vi "SetValueByArrayIndex.vi"(0 "VI Reference In":refnum<vi>, 2 "delimiter (>>)":string=">>", 5 "Control Path":string, 7 "Index Array":i32[](array[numeric]), 11 "Error In":errorcluster) -> (4 "VI Reference Out":refnum<vi>, 15 "Error Out":errorcluster)   [LabVIEW 2016, in "Drona.lvlib" / "ControlValue.lvlib" / "StimulusMCListbox.lvlib"]
doc: "Sets value(signaling) for the multi select multi column listbox control whose index values are specified. \n\nThe input control name is given as a string , incase of path, use delimiters inbetween the path."
uses:
  StimulusMCListbox.lvlib
  <vilib>/Utility/error.llb/Error Cluster From Error Code.vi
  <vilib>/ErrorRing/Error Ring.xnode
  Drona.lvlib
  Get/GetControlRef/GetControlRef.lvlib
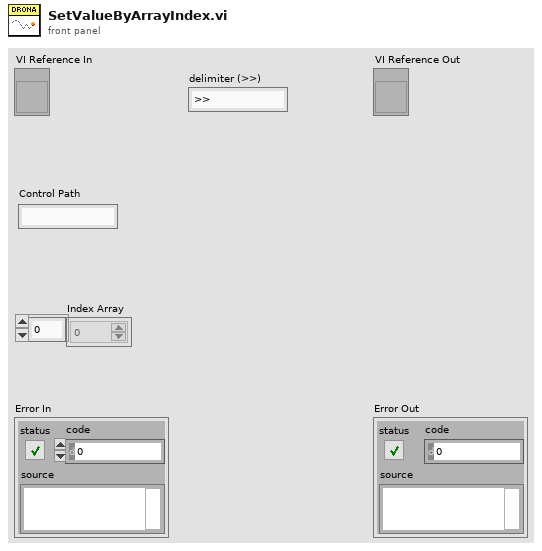
[diagram p1: front panel]
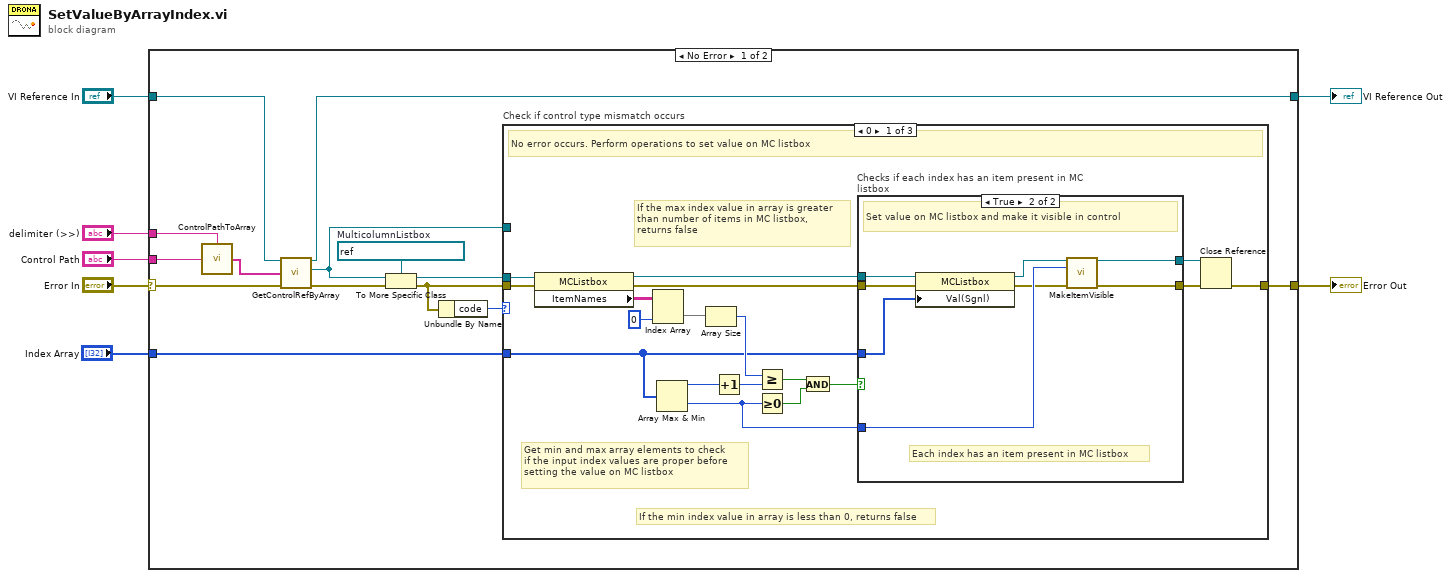
[diagram p0: block diagram]
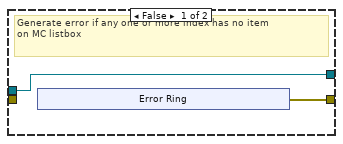
[diagram p2: hidden frame]
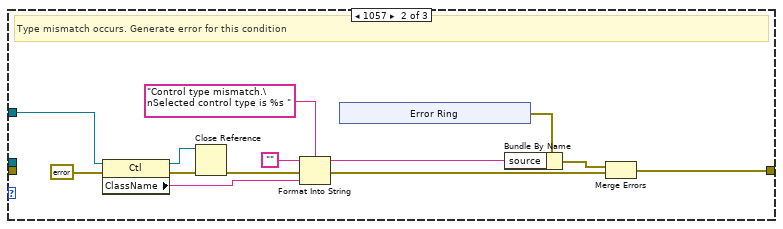
[diagram p3: hidden frame]
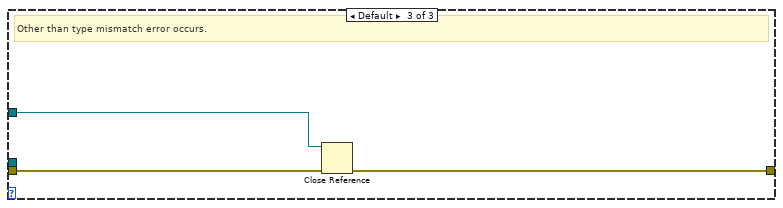
[diagram p4: hidden frame]
diagram:
  n1 = case shown="No Error" "Error In" {
    selector: "Error In" -> [w16 w77]
    tunnel: [w17 w77] -> w6
    tunnel: "VI Reference In" -> [w14 w76]
    tunnel: "Control Path" -> [w20 _]
    tunnel: "Index Array" -> [w11 _]
    tunnel: [w13 w76] -> w2
    tunnel: "delimiter (>>)" -> [w19 _]
    frame No Error {
      w21 = refnum<vi> refnum  # MulticolumnListbox
      n2 = call "ControlPathToArray.vi"("Control Name"=w20, "delimiter (>>)"=w19) -> ("Control Path"=w15:string[])
      n3 = call "GetControlRefByArray.vi"("VI Reference In"=w14, "Control Path"=w15, "error In"=w16) -> ("VI Reference Out"=w13:refnum<vi>, "Ctl Refnum"=w8:refnum<vi>, "error out"=w12:errorcluster)  [unwired: 10 in]
      n4 = To More Specific Class(target class=w21, reference=w8, error in=w12) -> (specific class reference=w18:refnum<vi>, error out=w10:errorcluster)
      n5 = Unbundle By Name(w10) -> ("code"=w9:i32)
      n6 = case "Check if control type mismatch occurs" shown="0" w9 {
        tunnel: w10 -> [w39 _ w75]
        tunnel: w18 -> [w35 _ _]
        tunnel: [w31 w55 w74] -> w17
        tunnel: w11 -> [w26 _ _]
        tunnel: w8 -> [_ w56 w73]
        frame 0 {
          # "If the min index value in array is less than 0, returns false"
          # "If the max index value in array is greater \nthan number of items in MC listbox, \nreturns false"
          # "Get min and max array elements to check \nif the input index values are proper before \nsetting the value on MC listbox"
          # "No error occurs. Perform operations to set value on MC listbox"
          n7 = property class="MCListbox"(reference=w35, error in=w39) -> (reference out=w34:refnum<vi>, error out=w36:errorcluster, "ItemNames"=w24:string[][])
          n8 = Index Array(array=w24, index (col)=0 ("disabled index (col)")) -> (element=w22:string[])  [unwired: 1 in]
          n9 = Array Max & Min(array=w26) -> (max value=w30:i32, min value=w28:i32)  [unwired: 2 out]
          n10 = Array Size(array=w22) -> (size(s)=w33:i32)
          n11 = Increment(x=w30) -> (x+1=w29:i32)
          n12 = Greater Or Equal?(x=w33, y=w29) -> (x >= y?=w27:bool)
          n13 = Greater Or Equal To 0?(x=w28) -> (x >= 0?=w25:bool)
          n14 = And(x=w27, y=w25) -> (x .and. y?=w32:bool)
          n15 = case "Checks if each index has an item present in MC listbox" shown="True" w32 {
            tunnel: [w40 w54] -> w38
            tunnel: [w41 w53] -> w37
            tunnel: w28 -> [_ w52]
            tunnel: w36 -> [_ w51]
            tunnel: w34 -> [w41 w49]
            tunnel: w26 -> [_ w48]
            frame False {
              # "Generate error if any one or more index has no item \non MC listbox"
              n16 = xnode "Error Ring"() -> ("error out"=w40:errorcluster)
            }
            frame True {
              # "Each index has an item present in MC listbox"
              # "Set value on MC listbox and make it visible in control"
              n17 = property class="MCListbox"(reference=w49, error in=w51, "Val(Sgnl)"=w48) -> (reference out=w47:refnum<vi>, error out=w50:errorcluster)
              n18 = call "MakeItemVisible.vi"("MC ListBox Ref In"=w47, "Item Index"=w52, "Error In"=w50) -> ("MC ListBox Ref Out"=w53:refnum<vi>, "Error Out"=w54:errorcluster)  [unwired: 11 in]
            }
          }
          n19 = Close Reference(reference=w37, error in (no error)=w38) -> (error out=w31:errorcluster)
        }
        frame 1057 {
          # "Type mismatch occurs. Generate error for this condition"
          n20 = property class="Ctl"(reference=w56, error in=errorcluster {"status"=FALSE, "code"=0, "source"=""} ("error out")) -> (reference out=w57:refnum<vi>, error out=w67:errorcluster, "ClassName"=w64:string)
          n21 = Close Reference(reference=w57, error in (no error)=w67) -> (error out=w58:errorcluster)
          n22 = Format Into String(format string="Control type mismatch.\nSelected control type is %s ", initial string="", error in=w58, w64) -> (resulting string=w61:string, error out=w59:errorcluster)
          n23 = xnode "Error Ring"() -> ("error out"=w62:errorcluster)
          n24 = Bundle By Name(cluster=w62, "source"=w61) -> (w60:errorcluster)
          n25 = Merge Errors(w60, w59) -> (w55:errorcluster)
        }
        frame Default {
          # "Other than type mismatch error occurs."
          n26 = Close Reference(reference=w73, error in (no error)=w75) -> (error out=w74:errorcluster)
        }
      }
    }
    frame Error {
    }
  }
  "Error Out" <- w6
  "VI Reference Out" <- w2
